vi "SIM Equal Times.vi"(4 "time 2":dbl, 5 "time 1":dbl) -> (0 "Time 2 <= Time 1?":bool, 1 "Time 2 == Time 1?":bool, 2 "Time 2 >= Time 1?":bool)   [LabVIEW 2010]
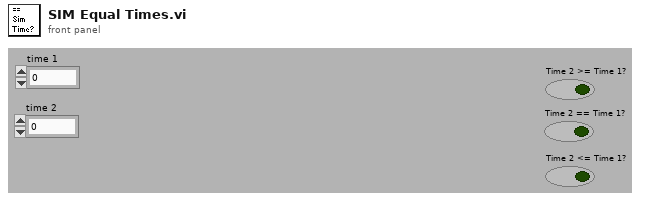
[diagram p1: front panel]
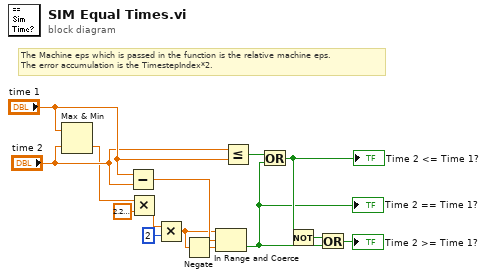
[diagram p0: block diagram]
diagram:
  # "The Machine eps which is passed in the function is the relative machine eps.\nThe error accumulation is the TimestepIndex*2."
  n1 = Max & Min(x="time 1", y="time 2") -> (min(x,y)=w8:dbl)  [unwired: 1 out]
  n2 = Subtract(x="time 1", y="time 2") -> (x-y=w4:dbl)
  n3 = Multiply(x=w8, y=2.220446049250313e-16) -> (x*y=w6:dbl)
  n4 = Multiply(x=w6, y=2 ("error accumulation")) -> (x*y=w1:dbl)
  n5 = Negate(x=w1) -> (-x=w2:dbl)
  n6 = In Range and Coerce(upper limit=w1, x=w4, lower limit=w2) -> (In Range?=w3:bool)  [unwired: 1 out]
  "Time 2 == Time 1?" <- w3
  n7 = Less Or Equal?(x="time 2", y="time 1") -> (x <= y?=w14:bool)
  n8 = Or(x=w14, y=w3) -> (x .or. y?=w11:bool)
  "Time 2 <= Time 1?" <- w11
  n9 = Not(x=w11) -> (.not. x?=w12:bool)
  n10 = Or(x=w12, y=w3) -> (x .or. y?=→"Time 2 >= Time 1?":bool)
